vi "Read Attributes.vi"(11 "Activate Microgrid Msg":refnum<class "Activate Microgrid Msg.lvclass">) -> (2 "Payload":cluster{"Data":variant})   [LabVIEW 2018, in "Remote Operation Abstract.lvlib" / "Activate Microgrid Msg.lvclass"]
uses:
  Activate Microgrid Msg.lvclass
  Activate Microgrid Msg.lvclass/Activate Microgrid Msg.ctl
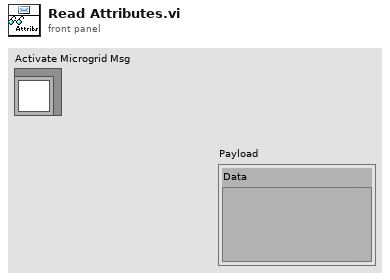
[diagram p1: front panel]
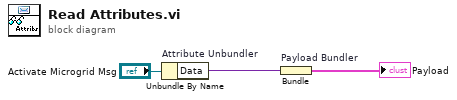
[diagram p0: block diagram]
diagram:
  n1 = Unbundle By Name "Attribute Unbundler"("Activate Microgrid Msg") -> ("Data"=w1:variant)
  n2 = Bundle "Payload Bundler"("Data"=w1) -> (→"Payload":cluster{"Data":variant})  [unwired: 1 in]
